vi "Update-status.vi"(6 "Status":T1, 8 "error in (no error)":errorcluster, 11 "Object ref in":T2) -> (0 "error out":errorcluster, 3 "Object ref out":T2)   [LabVIEW 2013, in "HardwareCharacterization.lvlib" / "HC-Main.lvclass"]
uses:
  HC-Main.lvclass
  Object-reference.ctl
  Application-status.ctl
  UI/Control-names.ctl
  HC-Main.lvclass/HC-Main.ctl
  Read UI.vi
  Write Status.vi
  UI/Set-control-string.vi
  UI/HC-UI.lvclass
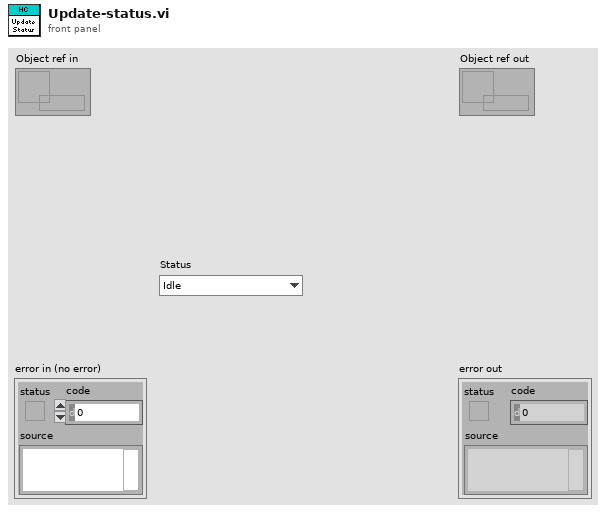
[diagram p1: front panel]
types:
  T1 = typedef "HardwareCharacterization.lvlib/HC-Main.lvclass/Application-status.ctl" = enum16{"Idle", "Initialized", "Configured", "Activated", "Started", "Paused", "Stopped", "Reset", "Error", "Exited"}
  T2 = typedef "HardwareCharacterization.lvlib/HC-Main.lvclass/Object-reference.ctl" = refnum<data-value>
  T3 = typedef "HardwareCharacterization.lvlib/HC-UI.lvclass/Control-names.ctl" = enum16{"Help", "Status", "Load configuration", "Save configuration", "Activate", "Start", "Stop", "Options"}
  T4 = typedef "HardwareCharacterization.lvlib/HC-UI.lvclass/Panes-reference.ctl" = refnum<data-value>
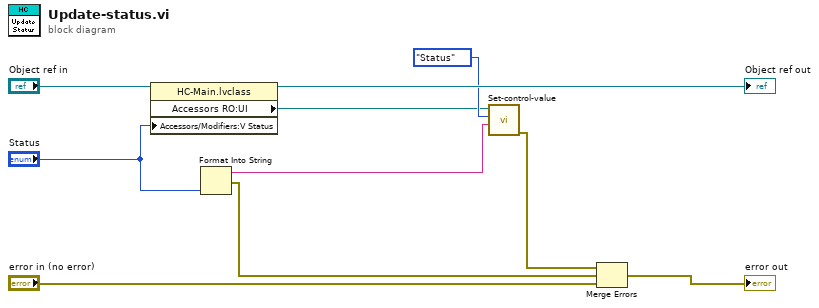
[diagram p0: block diagram]
diagram:
  n1 = property class="HC-Main.lvclass"(reference="Object ref in", "Accessors/Modifiers:V Status"="Status") -> (reference out=→"Object ref out":T2, "Accessors RO:UI"=w5:T4)  [unwired: 1 in, 1 out]
  n2 = Format Into String("Status") -> (resulting string=w3:string, error out=w4:errorcluster)  [unwired: 3 in]
  n3 = call-poly "Set-control-value.vi"("Value"=w3, "Control name"=Control-names."Status", "Panes in"=w5) -> ("error out"=w6:errorcluster)  [unwired: 7 in, 1 out]
  n4 = Merge Errors(w6, w4, "error in (no error)") -> (→"error out":errorcluster)
